vi "OSICS_Get_Settings_SWT-APC.vi"(7 "OSICS slot":i32=1, 8 "error in":errorcluster, 9 "Power Unit(dBm/mW)":bool, 10 "WL/F unit (nm/GHz)":bool, 11 "VISA IN":refnum<visa-resource-name>) -> (0 "error out":errorcluster, 2 "Laser Settings (Cluster)":T1, 3 "VISA OUT":refnum<visa-resource-name>)   [LabVIEW 2014, in "OSICS_LIB.lvlib"]
doc: "This Vi sets the WL/F unit, the Power unit and the operating mode from the OSICS SWT-APC module. Also, gets the following information in a cluster \"Laser Settings\":\nLaser State (ENABLE/DISABLE)\nWL/F (nm/GHz)\nPower (dBm/mW)\nPower and Current Limit reached (TRUE/FALSE)."
uses:
  OSICS_LIB.lvlib
panel:
  # "Basic Function to read the laser settings\nof the OSICS SWT APC"
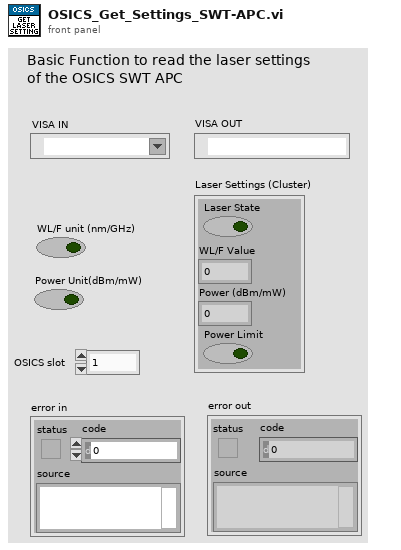
[diagram p1: front panel]
types:
  T1 = cluster{"Laser State":bool, "WL/F Value":dbl, "Power (dBm/mW)":dbl, "Power Limit":bool}
  T2 = cluster{"Laser State (DISABLED/ENABLED)":bool, "Current (mA)":dbl, "Current (mA)":dbl, "Laser State (DISABLED/ENABLED)":bool}
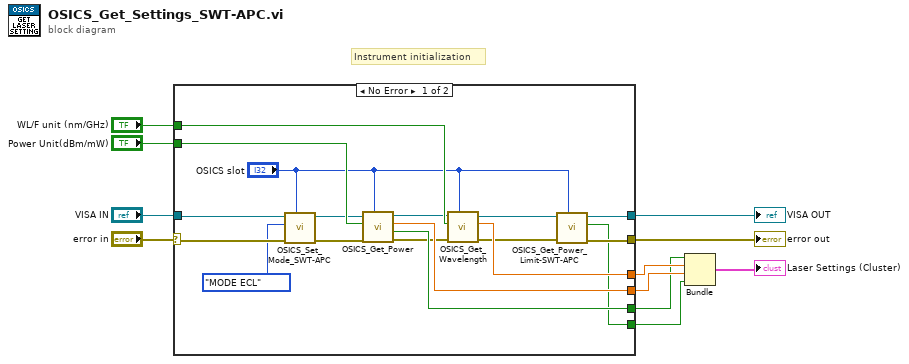
[diagram p0: block diagram]
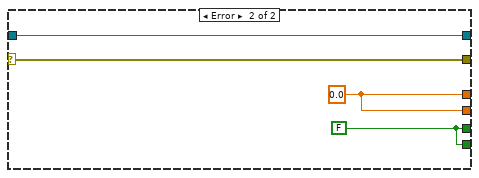
[diagram p2: hidden frame]
diagram:
  # "Instrument initialization"
  n1 = case shown="No Error" "error in" {
    selector: "error in" -> [w22 w32]
    tunnel: [w27 w30] -> w3
    tunnel: [w29 w31] -> w5
    tunnel: "WL/F unit (nm/GHz)" -> [w28 _]
    tunnel: [w24 w31] -> w4
    tunnel: "Power Unit(dBm/mW)" -> [w26 _]
    tunnel: "VISA IN" -> [w20 w33]
    tunnel: [w16 w33] -> w8
    tunnel: [w17 w32] -> w7
    tunnel: [w13 w30] -> w1
    frame No Error {
      n2 = call "OSICS_Set_Mode_SWT-APC.vi"("OSICS slot"="OSICS slot", "error in"=w22, "Mode"=enum16{"MODE ECL", "MODE SWT"}."MODE ECL", "VISA IN"=w20) -> ("error out"=w21:errorcluster, "VISA OUT"=w19:refnum<visa-resource-name>)  [unwired: 5 in, 1 out]
      n3 = call "OSICS_Get_Power.vi"("OSICS slot"="OSICS slot", "error in"=w21, "Power Unit(False: dBm)"=w26, "VISA IN"=w19) -> ("error out"=w23:errorcluster, "Laser State (False:Disabled)"=w27:bool, "Power (dBm/mW)"=w24:dbl, "VISA OUT"=w25:refnum<visa-resource-name>)  [unwired: 3 in, 1 out]
      n4 = call "OSICS_Get_Wavelength.vi"("OSICS slot"="OSICS slot", "error in"=w23, "WL/F unit (False:NM)"=w28, "VISA IN"=w25) -> ("error out"=w14:errorcluster, "WL/Frequency Value"=w29:dbl, "VISA OUT"=w15:refnum<visa-resource-name>)  [unwired: 4 in, 1 out]
      n5 = call "OSICS_Get_Power_Limit-SWT-APC.vi"("OSICS slot"="OSICS slot", "error in"=w14, "VISA IN"=w15) -> ("error out"=w17:errorcluster, "Power Limit"=w13:bool, "VISA OUT"=w16:refnum<visa-resource-name>)  [unwired: 5 in, 1 out]
    }
    frame Error {
      w31 = 0.0 ("Current (mA)")
      w30 = FALSE ("Laser State (DISABLED/ENABLED)")
    }
  }
  "VISA OUT" <- w8
  "error out" <- w7
  n6 = Bundle("Laser State (DISABLED/ENABLED)"=w3, "Current (mA)"=w5, "Current (mA)"=w4, "Laser State (DISABLED/ENABLED)"=w1) -> (→"Laser Settings (Cluster)":T2)  [unwired: 1 in]
